vi "PQresultErrorMessage.vi"(8 "error in (no error)":errorcluster, 10 "res":u64) -> (0 "error out":errorcluster, 1 "PQresultErrorMessage":string, 2 "res out":u64)   [LabVIEW 2019, in "libpqlv64.lvlib"]
doc: "Returns the error message associated with the command, or an empty string if there was no error."
uses:
  libpqlv64.lvlib
  libpq.dll
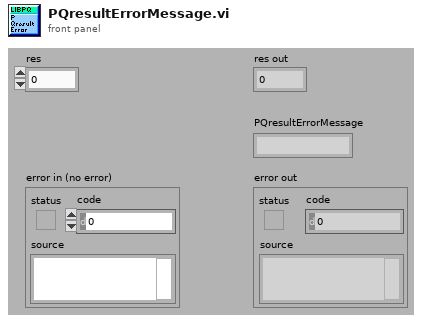
[diagram p1: front panel]
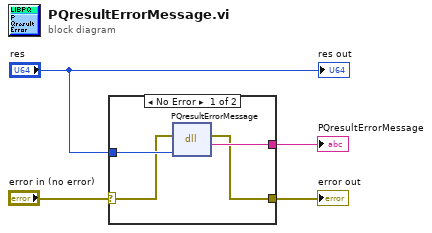
[diagram p0: block diagram]
diagram:
  n1 = case shown="No Error" "error in (no error)" {
    selector: "error in (no error)" -> [w6 w9]
    tunnel: [w5 w9] -> w3
    tunnel: [w8 _] -> w2
    tunnel: "res" -> [w7 _]
    frame No Error {
      n2 = dll-call lib="libpq.*" fn="PQresultErrorMessage"(error in=w6, "res"=w7) -> (error out=w5:errorcluster, "PQresultErrorMessage"=w8:string)  [unwired: 3 in, 1 out]
    }
    frame Error {
    }
  }
  "PQresultErrorMessage" <- w2
  "error out" <- w3
  "res out" <- "res"
